vi "Armed Response.vi"(8 "error in (no error)":errorcluster, 9 "Armed":bool, 10 "Sender":string, 11 "Pulse Controller in":refnum<class "Pulse Controller.lvclass">) -> (0 "error out":errorcluster, 3 "Pulse Controller out":refnum<class "Pulse Controller.lvclass">)   [LabVIEW 2018, in "Pulse Controller.lvclass"]
uses:
  Pulse Controller.lvclass
  C:/github/LabActor/Controllers/Process Controller/Process Controller.lvclass
  C:/Program Files/National Instruments/LabVIEW 2018/vi.lib/ActorFramework/Actor/Actor.lvclass
  Process Controller/Process Controller.lvclass/Process Controller.ctl
  Pulse Controller.lvclass/Pulse Controller.ctl
  <vilib>/ActorFramework/Actor/Actor.lvclass/Actor.ctl
  LabActor Messages/Update Armed Msg/Update Armed Msg.lvclass/Update Armed Msg.ctl
  <vilib>/ActorFramework/Message Enqueuer/Message Enqueuer.lvclass/Message Enqueuer.ctl
  Process Controller/Read Active measurements names.vi
  <vilib>/ActorFramework/Message Enqueuer/Enqueue.vi
  LabActor Messages/Update Armed Msg/Update Armed Msg.lvclass
  C:/Program Files/National Instruments/LabVIEW 2018/vi.lib/ActorFramework/Message/Message.lvclass
  <vilib>/ActorFramework/Message Priority Queue/Priority Enqueue.vi
  <vilib>/ActorFramework/Actor/Actor.lvclass
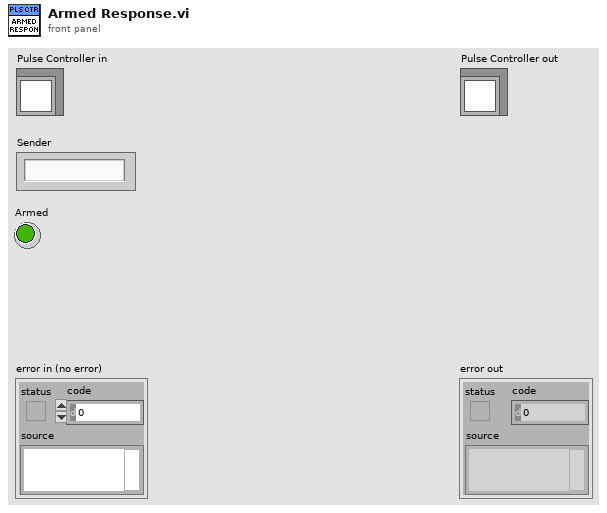
[diagram p1: front panel]
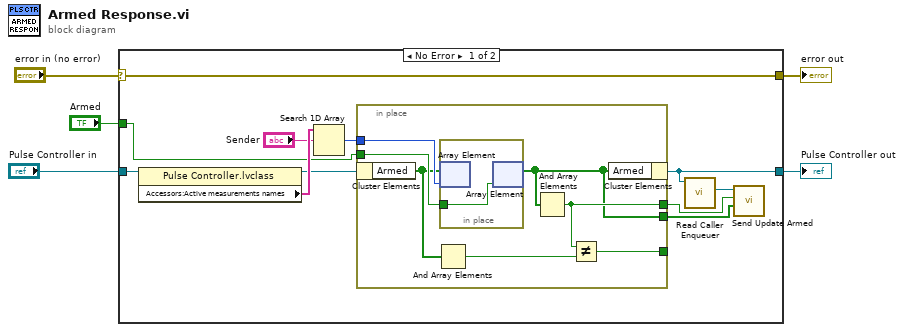
[diagram p0: block diagram]
diagram:
  n1 = case shown="No Error" "error in (no error)" {
    selector: "error in (no error)" -> [w15 w26]
    tunnel: [w15 w26] -> w4
    tunnel: [w8 w25] -> w2
    tunnel: "Pulse Controller in" -> [w16 w25]
    tunnel: "Armed" -> [w11 _]
    frame No Error {
      n2 = property class="Pulse Controller.lvclass"(reference=w16) -> (reference out=w10:refnum<class "Pulse Controller.lvclass">, "Accessors:Active measurements names"=w14:string[])  [unwired: 1 in, 1 out]
      n3 = Search 1D Array(1D array=w14, element="Sender") -> (index of element=w12:i32)  [unwired: 1 in]
      n4 = in-place {
        in-place-border: w12 -> [w23]
        in-place-border: w11 -> [w22]
        in-place-border: [w19] -> _
        in-place-border: [w18] -> w9
        in-place-border: [w17] -> w6
        n5 = in-place-cluster #1(w10) -> ("Armed"=w21:bool[])
        n6 = And Array Elements(Boolean array=w21) -> (logical AND=w20:bool)
        n7 = in-place {
          in-place-border: w22 -> [w24]
          n8 = in-place-array #2(w21, w23) -> ()  [unwired: 1 out]
          n9 = in-place-array #2(w24) -> (w17:bool[])  [unwired: 1 out]
        }
        n10 = And Array Elements(Boolean array=w17) -> (logical AND=w18:bool)
        n11 = Not Equal?(x=w18, y=w20) -> (x != y?=w19:bool)
        n12 = in-place-cluster #1("Armed"=w17) -> (w8:refnum<class "Pulse Controller.lvclass">)
      }
      n13 = call <vilib>:"Read Caller Enqueuer.vi"("Actor"=w8) -> ("Caller Enqueuer"=w7:refnum<class "Message Enqueuer.lvclass">)  [unwired: 10 in]
      n14 = call "Send Update Armed.vi"("Devices armed"=w6, "Armed"=w9, "Message Enqueuer"=w7) -> ()  [unwired: 7 in, 2 out]
    }
    frame Error {
    }
  }
  "error out" <- w4
  "Pulse Controller out" <- w2
